vi "Setup Motors.vi"   [LabVIEW 2014]
uses:
  <vilib>/Rock Robotics/SystemInterfaces/DIO/FPGA_DIOPWMChannel.ctl
  <vilib>/Rock Robotics/WPI/Joystick/WPI_JoystickDeviceEnum.ctl
  <vilib>/Rock Robotics/SystemInterfaces/Typedef/FPGA_TypedefDigitalModule.ctl
  <vilib>/Rock Robotics/SystemInterfaces/Typedef/FPGA_TypedefAnalogModule.ctl
  <vilib>/Rock Robotics/SystemInterfaces/AI/FPGA_AIChannel.ctl
  <vilib>/Rock Robotics/WPI/Solenoid/WPI_SolenoidChannel.ctl
  <vilib>/Rock Robotics/SystemInterfaces/AI/FPGA_AIGyroChannel.ctl
  <vilib>/Rock Robotics/SystemInterfaces/Typedef/FPGA_TypedefAnalogModuleForGyro.ctl
  <vilib>/Rock Robotics/SystemInterfaces/DIO/FPGA_DIOChannel.ctl
  <vilib>/Rock Robotics/WPI/SafetyOutput/WPI_SafetyOutputConfigMenu.ctl
  <vilib>/Rock Robotics/WPI/MotorControl/WPI_MotorControlOpen Jaguar.vi
  <vilib>/Rock Robotics/WPI/MotorControl/WPI_MotorControlOpen Talon.vi
  <vilib>/Rock Robotics/WPI/Solenoid/WPI_SolenoidOpenSingle.vi
  <vilib>/Rock Robotics/WPI/Switch/WPI_SwitchOpenLimit.vi
  <vilib>/Rock Robotics/WPI/Counter/WPI_CounterDigitalInputToDigitalSource.vi
  <vilib>/Rock Robotics/WPI/Counter/WPI_CounterOpen UpDown Mode.vi
  Global Variables.vi
types:
  T1 = typedef "FPGA_DIOChannel.ctl" = enum8{"DIO 0", "DIO 1", "DIO 2", "DIO 3", "DIO 4", "DIO 5", "DIO 6", "DIO 7", "DIO 8", "DIO 9", "DIO MXP 0", "DIO MXP 1", "DIO MXP 2", "DIO MXP 3", "DIO MXP 4", "DIO MXP 5", "DIO MXP 6", "DIO MXP 7", "DIO MXP 8", "DIO MXP 9", "DIO MXP 10", "DIO MXP 11", "DIO MXP 12", "DIO MXP 13", "DIO MXP 14", "DIO MXP 15", "Invalid"}
  T2 = typedef "WPI_SafetyOutputConfigMenu.ctl" = enum16{"Enable", "Disable"}
  T3 = typedef "FPGA_TypedefDigitalModule.ctl" = enum16{"Controller 1"}
  T4 = typedef "FPGA_TypedefAnalogModuleForGyro.ctl" = enum16{"Controller 1"}
  T5 = typedef "FPGA_AIGyroChannel.ctl" = enum8{"AI 0", "AI 1", "Invalid"}
  T6 = typedef "WPI_SolenoidChannel.ctl" = enum8{"Solenoid 0", "Solenoid 1", "Solenoid 2", "Solenoid 3", "Solenoid 4", "Solenoid 5", "Solenoid 6", "Solenoid 7", "Invalid"}
  T7 = typedef "FPGA_DIOPWMChannel.ctl" = enum8{"PWM 0", "PWM 1", "PWM 2", "PWM 3", "PWM 4", "PWM 5", "PWM 6", "PWM 7", "PWM 8", "PWM 9", "PWM MXP 0", "PWM MXP 1", "PWM MXP 2", "PWM MXP 3", "PWM MXP 4", "PWM MXP 5", "PWM MXP 6", "PWM MXP 7", "PWM MXP 8", "PWM MXP 9", "Invalid"}
  T8 = typedef "FPGA_AIChannel.ctl" = enum8{"AI 0", "AI 1", "AI 2", "AI 3", "AI MXP 0", "AI MXP 1", "AI MXP 2", "AI MXP 3", "Invalid"}
  T9 = typedef "FPGA_TypedefAnalogModule.ctl" = enum16{"Controller 1"}
  T10 = typedef "WPI_JoystickDeviceEnum.ctl" = enum16{"USB 0", "USB 1", "USB 2", "USB 3", "USB 4", "USB 5"}
  T11 = typedef "WPI_MotorControlDeviceRef.ctl" = cluster{"DeviceStatus":errorcluster, "Type":T12, "PWM":cluster{"Controller":T3, "PWM Channel":T7, "DeadBand":T13}, "CAN":cluster{"Device Number":u8, "Control Mode":T14, "Semaphore":T15, "Max Vout":dbl, "TalonSRX Control Mode":T16}, "Invert":bool, "TransformRef":T17, "InvTransformRef":T17}
  T12 = typedef "WPI_MotorControlType.ctl" = enum16{"PWM", "CAN", "CANTalonSRX"}
  T13 = typedef "WPI_PWMDeadband.ctl" = cluster{"Name":string, "maxPositivePwm":i32, "minPositivePwm":i32, "centerPwm":i32, "maxNegativePwm":i32, "minNegativePwm":i32, "angularRange":u16}
  T14 = typedef "WPI_CANJaguar_ControlMode.ctl" = enum8{"Percent VBus", "Current", "Speed", "Position", "Voltage"}
  T15 = typedef "Semaphore RefNum" = refnum<k1>
  T16 = typedef "WPI_CANTalonSRX_APIControlMode.ctl" = enum8{"Percent VBus", "Speed", "Position", "Slave", "Unchanged / Invalid"}
  T17 = typedef "WPI_PWMTransform_ConPane.ctl" = refnum<vi>
  T18 = typedef "WPI_GyroDevRef.ctl" = cluster{"DevStatus":errorcluster, "Analog Module":T9, "Analog Channel":T8, "Offset":dbl, "Gain (VoltsPerDegree/Second)":dbl}
  T19 = typedef "WPI_SolenoidDevRef.ctl" = cluster{"DevStatus":errorcluster, "Pneumatics Control Module":u8, "Forward Solenoid Channel":T6, "Reverse Solenoid Channel":T6}
  T20 = typedef "WPI_SwitchDevRef.ctl" = cluster{"DevStatus":errorcluster, "DIO Channel":T1, "Controller":T3, "CntIndex":T21, "Normally Closed":bool}
  T21 = typedef "FPGA_CounterCtrSystemIndex.ctl" = enum8{"Ctr 0", "Ctr 1", "Ctr 2", "Ctr 3", "Ctr 4", "Ctr 5", "Ctr 6", "Ctr 7", "Invalid"}
  T22 = typedef "WPI_AnalogChannelDevRef.ctl" = cluster{"DevStatus":errorcluster, "Controller":T9, "Analog Channel":T8}
  T23 = typedef "WPI_DigitalInputDevRef.ctl" = cluster{"DevStatus":errorcluster, "DIO Channel":T1, "Controller":T3}
  T24 = typedef "FPGA_CounterEncoderSourceConvertionLVSourceType.ctl" = cluster{"DevStatus":errorcluster, "AnalogTriggerMode?":bool, "DigitalMode":cluster{"Controller":T3, "DIO Channel":T25}, "AnalogTriggerMode":cluster{"AnalogTriggerIndex":T26, "OutputType":T27}}
  T25 = typedef "FPGA_DIODigitalSourceChannel.ctl" = enum8{"DIO 0", "DIO 1", "DIO 2", "DIO 3", "DIO 4", "DIO 5", "DIO 6", "DIO 7", "DIO 8", "DIO 9", "DIO MXP 0", "DIO MXP 1", "DIO MXP 2", "DIO MXP 3", "DIO MXP 4", "DIO MXP 5", "DIO MXP 6", "DIO MXP 7", "DIO MXP 8", "DIO MXP 9", "DIO MXP 10", "DIO MXP 11", "DIO MXP 12", "DIO MXP 13", "DIO MXP 14", "DIO MXP 15", "Disabled"}
  T26 = typedef "FPGA_AnalogTriggerIndex.ctl" = enum8{"Trig 0", "Trig 1", "Trig 2", "Trig 3", "Trig 4", "Trig 5", "Trig 6", "Trig 7", "Invalid"}
  T27 = typedef "FPGA_AnalogTriggerOutType.ctl" = enum16{"InWindow", "TriggerState", "Rising", "Falling"}
  T28 = typedef "WPI_EncoderDevRef.ctl" = cluster{"DevStatus":errorcluster, "EncoderIndex":T29, "CounterIndex":T21, "DistancePerCount":dbl, "Decoding Type":T30}
  T29 = typedef "FPGA_EncoderIdx.ctl" = enum8{"Enc 0", "Enc 1", "Enc 2", "Enc 3", "Enc 4", "Enc 5", "Enc 6", "Enc 7", "Invalid"}
  T30 = typedef "WPI_EncoderType.ctl" = enum16{"1x", "2x", "4x"}
  T31 = typedef "WPI_CounterDevRef.ctl" = cluster{"DevStatus":errorcluster, "CntIndex":T21}
  T32 = typedef "WPI_JoystickDevRef.ctl" = cluster{"Device":T10}
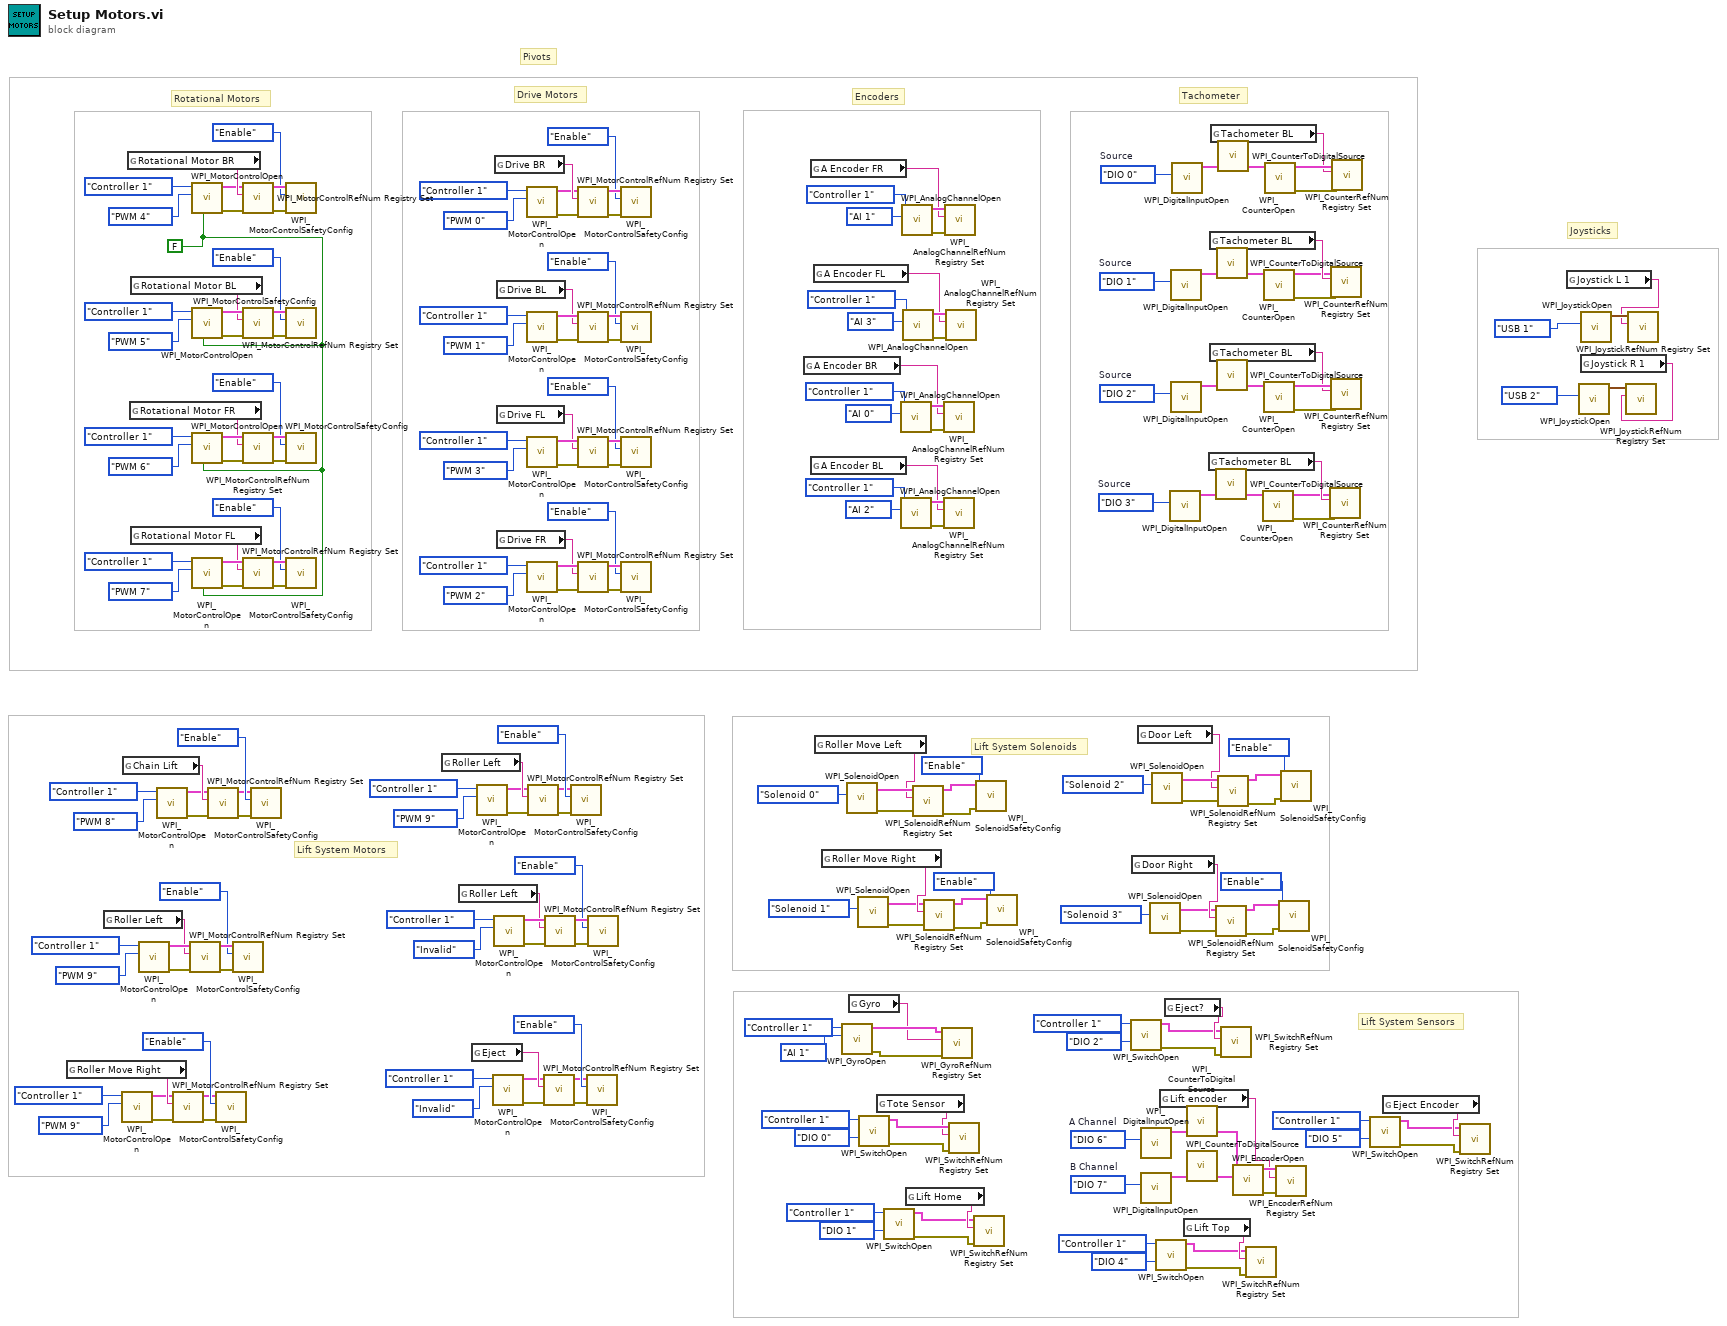
[diagram p0: block diagram]
diagram:
  w2 = FPGA_DIOChannel."DIO 3"  # Source
  w11 = FPGA_DIOChannel."DIO 2"  # Source
  w14 = FPGA_DIOChannel."DIO 1"  # Source
  w23 = FPGA_DIOChannel."DIO 0"  # Source
  w25 = FALSE ("Invert")
  w34 = FPGA_DIOChannel."DIO 7"  # B Channel
  w33 = FPGA_DIOChannel."DIO 6"  # A Channel
  # "Tachometer"
  # "Lift System Sensors"
  # "Lift System Solenoids"
  # "Lift System Motors"
  # "Encoders"
  # "Joysticks"
  # "Pivots"
  # "Rotational Motors"
  # "Drive Motors"
  n1 = global read "Global Variables.vi" "Roller Move Right"() -> (w123:string)
  n2 = global read "Global Variables.vi" "Roller Left"() -> (w126:string)
  n3 = call-poly <vilib>:"WPI_MotorControlOpen.vi"("PWM Channel"=FPGA_DIOPWMChannel."PWM 9", "Controller"=FPGA_TypedefDigitalModule."Controller 1") -> ("error out"=w118:errorcluster, "MotorControlDeviceRef"=w117:T11)  [unwired: 8 in]
  n4 = global read "Global Variables.vi" "Chain Lift"() -> (w139:string)
  n5 = global read "Global Variables.vi" "Rotational Motor BR"() -> (w193:string)
  n6 = global read "Global Variables.vi" "Rotational Motor FR"() -> (w167:string)
  n7 = global read "Global Variables.vi" "Rotational Motor BL"() -> (w168:string)
  n8 = global read "Global Variables.vi" "Rotational Motor FL"() -> (w166:string)
  n9 = call-poly <vilib>:"WPI_MotorControlOpen.vi"("PWM Channel"=FPGA_DIOPWMChannel."PWM 9", "Controller"=FPGA_TypedefDigitalModule."Controller 1") -> ("error out"=w131:errorcluster, "MotorControlDeviceRef"=w132:T11)  [unwired: 8 in]
  n10 = call-poly <vilib>:"WPI_MotorControlOpen.vi"("PWM Channel"=FPGA_DIOPWMChannel."PWM 8", "Controller"=FPGA_TypedefDigitalModule."Controller 1") -> ("error out"=w134:errorcluster, "MotorControlDeviceRef"=w133:T11)  [unwired: 8 in]
  n11 = call <vilib>:"WPI_MotorControlRefNum Registry Set.vi"("error in (no error)"=w118, "refnum name"=w123, "MotorControlDevRef"=w117) -> ("error out"=w120:errorcluster, "MotorControlDevRef"=w119:T11)  [unwired: 7 in]
  n12 = call <vilib>:"WPI_MotorControlRefNum Registry Set.vi"("error in (no error)"=w131, "refnum name"=w126, "MotorControlDevRef"=w132) -> ("error out"=w129:errorcluster, "MotorControlDevRef"=w130:T11)  [unwired: 7 in]
  n13 = call-poly <vilib>:"WPI_MotorControlOpen.vi"("Invert"=w25, "PWM Channel"=FPGA_DIOPWMChannel."PWM 4", "Controller"=FPGA_TypedefDigitalModule."Controller 1") -> ("error out"=w191:errorcluster, "MotorControlDeviceRef"=w192:T11)  [unwired: 7 in]
  n14 = call-poly <vilib>:"WPI_MotorControlOpen.vi"("Invert"=w25, "PWM Channel"=FPGA_DIOPWMChannel."PWM 5", "Controller"=FPGA_TypedefDigitalModule."Controller 1") -> ("error out"=w185:errorcluster, "MotorControlDeviceRef"=w186:T11)  [unwired: 7 in]
  n15 = call-poly <vilib>:"WPI_MotorControlOpen.vi"("Invert"=w25, "PWM Channel"=FPGA_DIOPWMChannel."PWM 6", "Controller"=FPGA_TypedefDigitalModule."Controller 1") -> ("error out"=w179:errorcluster, "MotorControlDeviceRef"=w180:T11)  [unwired: 7 in]
  n16 = call-poly <vilib>:"WPI_MotorControlOpen.vi"("Invert"=w25, "PWM Channel"=FPGA_DIOPWMChannel."PWM 7", "Controller"=FPGA_TypedefDigitalModule."Controller 1") -> ("error out"=w173:errorcluster, "MotorControlDeviceRef"=w174:T11)  [unwired: 7 in]
  n17 = call <vilib>:"WPI_MotorControlRefNum Registry Set.vi"("error in (no error)"=w134, "refnum name"=w139, "MotorControlDevRef"=w133) -> ("error out"=w136:errorcluster, "MotorControlDevRef"=w135:T11)  [unwired: 7 in]
  n18 = call <vilib>:"WPI_MotorControlSafetyConfig.vi"("error in (no error)"=w120, "mode"=WPI_SafetyOutputConfigMenu."Enable", "MotorControlDevRef"=w119) -> ()  [unwired: 7 in, 2 out]
  n19 = call <vilib>:"WPI_MotorControlSafetyConfig.vi"("error in (no error)"=w129, "mode"=WPI_SafetyOutputConfigMenu."Enable", "MotorControlDevRef"=w130) -> ()  [unwired: 7 in, 2 out]
  n20 = call <vilib>:"WPI_MotorControlRefNum Registry Set.vi"("error in (no error)"=w191, "refnum name"=w193, "MotorControlDevRef"=w192) -> ("error out"=w189:errorcluster, "MotorControlDevRef"=w190:T11)  [unwired: 7 in]
  n21 = call <vilib>:"WPI_MotorControlRefNum Registry Set.vi"("error in (no error)"=w185, "refnum name"=w168, "MotorControlDevRef"=w186) -> ("error out"=w183:errorcluster, "MotorControlDevRef"=w184:T11)  [unwired: 7 in]
  n22 = call <vilib>:"WPI_MotorControlRefNum Registry Set.vi"("error in (no error)"=w179, "refnum name"=w167, "MotorControlDevRef"=w180) -> ("error out"=w177:errorcluster, "MotorControlDevRef"=w178:T11)  [unwired: 7 in]
  n23 = call <vilib>:"WPI_MotorControlRefNum Registry Set.vi"("error in (no error)"=w173, "refnum name"=w166, "MotorControlDevRef"=w174) -> ("error out"=w171:errorcluster, "MotorControlDevRef"=w172:T11)  [unwired: 7 in]
  n24 = call <vilib>:"WPI_MotorControlSafetyConfig.vi"("error in (no error)"=w136, "mode"=WPI_SafetyOutputConfigMenu."Enable", "MotorControlDevRef"=w135) -> ()  [unwired: 7 in, 2 out]
  n25 = call <vilib>:"WPI_MotorControlSafetyConfig.vi"("error in (no error)"=w189, "mode"=WPI_SafetyOutputConfigMenu."Enable", "MotorControlDevRef"=w190) -> ()  [unwired: 7 in, 2 out]
  n26 = call <vilib>:"WPI_MotorControlSafetyConfig.vi"("error in (no error)"=w183, "mode"=WPI_SafetyOutputConfigMenu."Enable", "MotorControlDevRef"=w184) -> ()  [unwired: 7 in, 2 out]
  n27 = call <vilib>:"WPI_MotorControlSafetyConfig.vi"("error in (no error)"=w177, "mode"=WPI_SafetyOutputConfigMenu."Enable", "MotorControlDevRef"=w178) -> ()  [unwired: 7 in, 2 out]
  n28 = call <vilib>:"WPI_MotorControlSafetyConfig.vi"("error in (no error)"=w171, "mode"=WPI_SafetyOutputConfigMenu."Enable", "MotorControlDevRef"=w172) -> ()  [unwired: 7 in, 2 out]
  n29 = global read "Global Variables.vi" "Roller Left"() -> (w115:string)
  n30 = global read "Global Variables.vi" "Roller Left"() -> (w102:string)
  n31 = global read "Global Variables.vi" "Eject"() -> (w99:string)
  n32 = call-poly <vilib>:"WPI_MotorControlOpen.vi"("PWM Channel"=FPGA_DIOPWMChannel."PWM 9", "Controller"=FPGA_TypedefDigitalModule."Controller 1") -> ("error out"=w110:errorcluster, "MotorControlDeviceRef"=w109:T11)  [unwired: 8 in]
  n33 = call-poly <vilib>:"WPI_MotorControlOpen.vi"("PWM Channel"=FPGA_DIOPWMChannel."Invalid", "Controller"=FPGA_TypedefDigitalModule."Controller 1") -> ("error out"=w94:errorcluster, "MotorControlDeviceRef"=w93:T11)  [unwired: 8 in]
  n34 = call-poly <vilib>:"WPI_MotorControlOpen.vi"("PWM Channel"=FPGA_DIOPWMChannel."Invalid", "Controller"=FPGA_TypedefDigitalModule."Controller 1") -> ("error out"=w107:errorcluster, "MotorControlDeviceRef"=w108:T11)  [unwired: 8 in]
  n35 = global read "Global Variables.vi" "Drive BR"() -> (w230:string)
  n36 = global read "Global Variables.vi" "Drive BL"() -> (w205:string)
  n37 = global read "Global Variables.vi" "Drive FL"() -> (w204:string)
  n38 = global read "Global Variables.vi" "Drive FR"() -> (w203:string)
  n39 = call-poly <vilib>:"WPI_MotorControlOpen.vi"("PWM Channel"=FPGA_DIOPWMChannel."PWM 0", "Controller"=FPGA_TypedefDigitalModule."Controller 1") -> ("error out"=w228:errorcluster, "MotorControlDeviceRef"=w229:T11)  [unwired: 8 in]
  n40 = call-poly <vilib>:"WPI_MotorControlOpen.vi"("PWM Channel"=FPGA_DIOPWMChannel."PWM 1", "Controller"=FPGA_TypedefDigitalModule."Controller 1") -> ("error out"=w222:errorcluster, "MotorControlDeviceRef"=w223:T11)  [unwired: 8 in]
  n41 = call-poly <vilib>:"WPI_MotorControlOpen.vi"("PWM Channel"=FPGA_DIOPWMChannel."PWM 3", "Controller"=FPGA_TypedefDigitalModule."Controller 1") -> ("error out"=w216:errorcluster, "MotorControlDeviceRef"=w217:T11)  [unwired: 8 in]
  n42 = call-poly <vilib>:"WPI_MotorControlOpen.vi"("PWM Channel"=FPGA_DIOPWMChannel."PWM 2", "Controller"=FPGA_TypedefDigitalModule."Controller 1") -> ("error out"=w210:errorcluster, "MotorControlDeviceRef"=w211:T11)  [unwired: 8 in]
  n43 = call <vilib>:"WPI_MotorControlRefNum Registry Set.vi"("error in (no error)"=w110, "refnum name"=w115, "MotorControlDevRef"=w109) -> ("error out"=w112:errorcluster, "MotorControlDevRef"=w111:T11)  [unwired: 7 in]
  n44 = call <vilib>:"WPI_MotorControlRefNum Registry Set.vi"("error in (no error)"=w94, "refnum name"=w99, "MotorControlDevRef"=w93) -> ("error out"=w96:errorcluster, "MotorControlDevRef"=w95:T11)  [unwired: 7 in]
  n45 = call <vilib>:"WPI_MotorControlRefNum Registry Set.vi"("error in (no error)"=w107, "refnum name"=w102, "MotorControlDevRef"=w108) -> ("error out"=w105:errorcluster, "MotorControlDevRef"=w106:T11)  [unwired: 7 in]
  n46 = call <vilib>:"WPI_MotorControlSafetyConfig.vi"("error in (no error)"=w112, "mode"=WPI_SafetyOutputConfigMenu."Enable", "MotorControlDevRef"=w111) -> ()  [unwired: 7 in, 2 out]
  n47 = call <vilib>:"WPI_MotorControlRefNum Registry Set.vi"("error in (no error)"=w228, "refnum name"=w230, "MotorControlDevRef"=w229) -> ("error out"=w226:errorcluster, "MotorControlDevRef"=w227:T11)  [unwired: 7 in]
  n48 = call <vilib>:"WPI_MotorControlRefNum Registry Set.vi"("error in (no error)"=w222, "refnum name"=w205, "MotorControlDevRef"=w223) -> ("error out"=w220:errorcluster, "MotorControlDevRef"=w221:T11)  [unwired: 7 in]
  n49 = call <vilib>:"WPI_MotorControlRefNum Registry Set.vi"("error in (no error)"=w216, "refnum name"=w204, "MotorControlDevRef"=w217) -> ("error out"=w214:errorcluster, "MotorControlDevRef"=w215:T11)  [unwired: 7 in]
  n50 = call <vilib>:"WPI_MotorControlRefNum Registry Set.vi"("error in (no error)"=w210, "refnum name"=w203, "MotorControlDevRef"=w211) -> ("error out"=w208:errorcluster, "MotorControlDevRef"=w209:T11)  [unwired: 7 in]
  n51 = call <vilib>:"WPI_MotorControlSafetyConfig.vi"("error in (no error)"=w96, "mode"=WPI_SafetyOutputConfigMenu."Enable", "MotorControlDevRef"=w95) -> ()  [unwired: 7 in, 2 out]
  n52 = call <vilib>:"WPI_MotorControlSafetyConfig.vi"("error in (no error)"=w105, "mode"=WPI_SafetyOutputConfigMenu."Enable", "MotorControlDevRef"=w106) -> ()  [unwired: 7 in, 2 out]
  n53 = call <vilib>:"WPI_MotorControlSafetyConfig.vi"("error in (no error)"=w226, "mode"=WPI_SafetyOutputConfigMenu."Enable", "MotorControlDevRef"=w227) -> ()  [unwired: 7 in, 2 out]
  n54 = call <vilib>:"WPI_MotorControlSafetyConfig.vi"("error in (no error)"=w220, "mode"=WPI_SafetyOutputConfigMenu."Enable", "MotorControlDevRef"=w221) -> ()  [unwired: 7 in, 2 out]
  n55 = call <vilib>:"WPI_MotorControlSafetyConfig.vi"("error in (no error)"=w214, "mode"=WPI_SafetyOutputConfigMenu."Enable", "MotorControlDevRef"=w215) -> ()  [unwired: 7 in, 2 out]
  n56 = call <vilib>:"WPI_MotorControlSafetyConfig.vi"("error in (no error)"=w208, "mode"=WPI_SafetyOutputConfigMenu."Enable", "MotorControlDevRef"=w209) -> ()  [unwired: 7 in, 2 out]
  n57 = global read "Global Variables.vi" "A Encoder BR"() -> (w142:string)
  n58 = global read "Global Variables.vi" "A Encoder FR"() -> (w144:string)
  n59 = global read "Global Variables.vi" "A Encoder BL"() -> (w143:string)
  n60 = global read "Global Variables.vi" "A Encoder FL"() -> (w141:string)
  n61 = global read "Global Variables.vi" "Roller Move Left"() -> (w87:string)
  n62 = global read "Global Variables.vi" "Roller Move Right"() -> (w86:string)
  n63 = call <vilib>:"WPI_GyroOpen.vi"("Analog Channel"=FPGA_AIGyroChannel."AI 1", "Controller"=FPGA_TypedefAnalogModuleForGyro."Controller 1") -> ("error out"=w67:errorcluster, "GyroDevRef"=w68:T18)  [unwired: 7 in, 1 out]
  n64 = call-poly <vilib>:"WPI_SolenoidOpen.vi"("Solenoid Channel"=WPI_SolenoidChannel."Solenoid 0") -> ("error out"=w89:errorcluster, "SolenoidDevRef"=w90:T19)  [unwired: 9 in]
  n65 = global read "Global Variables.vi" "Gyro"() -> (w64:string)
  n66 = call-poly <vilib>:"WPI_SolenoidOpen.vi"("Solenoid Channel"=WPI_SolenoidChannel."Solenoid 1") -> ("error out"=w84:errorcluster, "SolenoidDevRef"=w83:T19)  [unwired: 9 in]
  n67 = call-poly <vilib>:"WPI_SwitchOpen.vi"("DIO Channel"=FPGA_DIOChannel."DIO 0", "Controller"=FPGA_TypedefDigitalModule."Controller 1") -> ("error out"=w62:errorcluster, "SwitchDevRef"=w63:T20)  [unwired: 8 in]
  n68 = global read "Global Variables.vi" "Tote Sensor"() -> (w59:string)
  n69 = call-poly <vilib>:"WPI_SwitchOpen.vi"("DIO Channel"=FPGA_DIOChannel."DIO 1", "Controller"=FPGA_TypedefDigitalModule."Controller 1") -> ("error out"=w55:errorcluster, "SwitchDevRef"=w54:T20)  [unwired: 8 in]
  n70 = call <vilib>:"WPI_AnalogChannelOpen.vi"("Analog Channel"=FPGA_AIChannel."AI 0", "Controller"=FPGA_TypedefAnalogModule."Controller 1") -> ("error out"=w151:errorcluster, "AIDeviceRef"=w152:T22)  [unwired: 8 in]
  n71 = call <vilib>:"WPI_AnalogChannelOpen.vi"("Analog Channel"=FPGA_AIChannel."AI 2", "Controller"=FPGA_TypedefAnalogModule."Controller 1") -> ("error out"=w147:errorcluster, "AIDeviceRef"=w148:T22)  [unwired: 8 in]
  n72 = call <vilib>:"WPI_AnalogChannelOpen.vi"("Analog Channel"=FPGA_AIChannel."AI 1", "Controller"=FPGA_TypedefAnalogModule."Controller 1") -> ("error out"=w159:errorcluster, "AIDeviceRef"=w160:T22)  [unwired: 8 in]
  n73 = call <vilib>:"WPI_AnalogChannelOpen.vi"("Analog Channel"=FPGA_AIChannel."AI 3", "Controller"=FPGA_TypedefAnalogModule."Controller 1") -> ("error out"=w155:errorcluster, "AIDeviceRef"=w156:T22)  [unwired: 8 in]
  n74 = global read "Global Variables.vi" "Lift Home"() -> (w58:string)
  n75 = call <vilib>:"WPI_SolenoidRefNum Registry Set.vi"("error in (no error)"=w89, "refnum name"=w87, "SolenoidDevRef"=w90) -> ("error out"=w91:errorcluster, "SolenoidDevRef"=w92:T19)  [unwired: 7 in]
  n76 = call <vilib>:"WPI_SolenoidRefNum Registry Set.vi"("error in (no error)"=w84, "refnum name"=w86, "SolenoidDevRef"=w83) -> ("error out"=w82:errorcluster, "SolenoidDevRef"=w81:T19)  [unwired: 7 in]
  n77 = call <vilib>:"WPI_GyroRefNum Registry Set.vi"("error in (no error)"=w67, "refnum name"=w64, "GyroDevRef"=w68) -> ()  [unwired: 7 in, 2 out]
  n78 = call <vilib>:"WPI_AnalogChannelRefNum Registry Set.vi"("error in (no error)"=w151, "refnum name"=w142, "AIDeviceRef"=w152) -> ()  [unwired: 7 in, 2 out]
  n79 = call <vilib>:"WPI_AnalogChannelRefNum Registry Set.vi"("error in (no error)"=w147, "refnum name"=w143, "AIDeviceRef"=w148) -> ()  [unwired: 7 in, 2 out]
  n80 = call <vilib>:"WPI_AnalogChannelRefNum Registry Set.vi"("error in (no error)"=w159, "refnum name"=w144, "AIDeviceRef"=w160) -> ()  [unwired: 7 in, 2 out]
  n81 = call <vilib>:"WPI_AnalogChannelRefNum Registry Set.vi"("error in (no error)"=w155, "refnum name"=w141, "AIDeviceRef"=w156) -> ()  [unwired: 7 in, 2 out]
  n82 = call <vilib>:"WPI_SwitchRefNum Registry Set.vi"("error in (no error)"=w62, "refnum name"=w59, "SwitchDevRef"=w63) -> ()  [unwired: 7 in, 2 out]
  n83 = call <vilib>:"WPI_SwitchRefNum Registry Set.vi"("error in (no error)"=w55, "refnum name"=w58, "SwitchDevRef"=w54) -> ()  [unwired: 7 in, 2 out]
  n84 = call <vilib>:"WPI_SolenoidSafetyConfig.vi"("error in (no error)"=w91, "mode"=WPI_SafetyOutputConfigMenu."Enable", "SolenoidDevRef"=w92) -> ()  [unwired: 7 in, 2 out]
  n85 = call <vilib>:"WPI_SolenoidSafetyConfig.vi"("error in (no error)"=w82, "mode"=WPI_SafetyOutputConfigMenu."Enable", "SolenoidDevRef"=w81) -> ()  [unwired: 7 in, 2 out]
  n86 = call-poly <vilib>:"WPI_SwitchOpen.vi"("DIO Channel"=FPGA_DIOChannel."DIO 2", "Controller"=FPGA_TypedefDigitalModule."Controller 1") -> ("error out"=w45:errorcluster, "SwitchDevRef"=w44:T20)  [unwired: 8 in]
  n87 = global read "Global Variables.vi" "Door Right"() -> (w74:string)
  n88 = global read "Global Variables.vi" "Door Left"() -> (w75:string)
  n89 = call <vilib>:"WPI_DigitalInputOpen.vi"("DIO Channel"=w33) -> ("DigitalInputDevRef"=w30:T23)  [unwired: 2 in, 8 out]
  n90 = call <vilib>:"WPI_DigitalInputOpen.vi"("DIO Channel"=w34) -> ("DigitalInputDevRef"=w31:T23)  [unwired: 2 in, 8 out]
  n91 = call-poly <vilib>:"WPI_SolenoidOpen.vi"("Solenoid Channel"=WPI_SolenoidChannel."Solenoid 3") -> ("error out"=w72:errorcluster, "SolenoidDevRef"=w71:T19)  [unwired: 9 in]
  n92 = call-poly <vilib>:"WPI_SolenoidOpen.vi"("Solenoid Channel"=WPI_SolenoidChannel."Solenoid 2") -> ("error out"=w77:errorcluster, "SolenoidDevRef"=w78:T19)  [unwired: 9 in]
  n93 = call-poly <vilib>:"WPI_SwitchOpen.vi"("DIO Channel"=FPGA_DIOChannel."DIO 4", "Controller"=FPGA_TypedefDigitalModule."Controller 1") -> ("error out"=w50:errorcluster, "SwitchDevRef"=w49:T20)  [unwired: 8 in]
  n94 = global read "Global Variables.vi" "Lift encoder"() -> (w26:string)
  n95 = global read "Global Variables.vi" "Eject?"() -> (w48:string)
  n96 = call <vilib>:"WPI_DigitalInputOpen.vi"("DIO Channel"=w2) -> ("DigitalInputDevRef"=w3:T23)  [unwired: 2 in, 8 out]
  n97 = call <vilib>:"WPI_DigitalInputOpen.vi"("DIO Channel"=w14) -> ("DigitalInputDevRef"=w15:T23)  [unwired: 2 in, 8 out]
  n98 = call <vilib>:"WPI_DigitalInputOpen.vi"("DIO Channel"=w11) -> ("DigitalInputDevRef"=w10:T23)  [unwired: 2 in, 8 out]
  n99 = call <vilib>:"WPI_DigitalInputOpen.vi"("DIO Channel"=w23) -> ("DigitalInputDevRef"=w22:T23)  [unwired: 2 in, 8 out]
  n100 = global read "Global Variables.vi" "Lift Top"() -> (w53:string)
  n101 = call-poly <vilib>:"WPI_CounterToDigitalSource.vi"("DigitalInputDevRef"=w30) -> ("Digital Source"=w29:T24)  [unwired: 6 out]
  n102 = call-poly <vilib>:"WPI_CounterToDigitalSource.vi"("DigitalInputDevRef"=w31) -> ("Digital Source"=w32:T24)  [unwired: 6 out]
  n103 = global read "Global Variables.vi" "Tachometer BL"() -> (w6:string)
  n104 = global read "Global Variables.vi" "Tachometer BL"() -> (w18:string)
  n105 = global read "Global Variables.vi" "Tachometer BL"() -> (w7:string)
  n106 = global read "Global Variables.vi" "Tachometer BL"() -> (w19:string)
  n107 = call-poly <vilib>:"WPI_CounterToDigitalSource.vi"("DigitalInputDevRef"=w3) -> ("Digital Source"=w1:T24)  [unwired: 6 out]
  n108 = call <vilib>:"WPI_SolenoidRefNum Registry Set.vi"("error in (no error)"=w72, "refnum name"=w74, "SolenoidDevRef"=w71) -> ("error out"=w70:errorcluster, "SolenoidDevRef"=w69:T19)  [unwired: 7 in]
  n109 = call-poly <vilib>:"WPI_CounterToDigitalSource.vi"("DigitalInputDevRef"=w15) -> ("Digital Source"=w13:T24)  [unwired: 6 out]
  n110 = call-poly <vilib>:"WPI_CounterToDigitalSource.vi"("DigitalInputDevRef"=w10) -> ("Digital Source"=w12:T24)  [unwired: 6 out]
  n111 = call-poly <vilib>:"WPI_CounterToDigitalSource.vi"("DigitalInputDevRef"=w22) -> ("Digital Source"=w24:T24)  [unwired: 6 out]
  n112 = call <vilib>:"WPI_SolenoidRefNum Registry Set.vi"("error in (no error)"=w77, "refnum name"=w75, "SolenoidDevRef"=w78) -> ("error out"=w79:errorcluster, "SolenoidDevRef"=w80:T19)  [unwired: 7 in]
  n113 = call <vilib>:"WPI_SwitchRefNum Registry Set.vi"("error in (no error)"=w45, "refnum name"=w48, "SwitchDevRef"=w44) -> ()  [unwired: 7 in, 2 out]
  n114 = call <vilib>:"WPI_EncoderOpen.vi"("BSource"=w32, "ASource"=w29) -> ("error out"=w28:errorcluster, "EncoderDevRef"=w27:T28)  [unwired: 6 in, 2 out]
  n115 = call <vilib>:"WPI_SwitchRefNum Registry Set.vi"("error in (no error)"=w50, "refnum name"=w53, "SwitchDevRef"=w49) -> ()  [unwired: 7 in, 2 out]
  n116 = call-poly <vilib>:"WPI_CounterOpen.vi"("Up Source"=w1) -> ("error out"=w5:errorcluster, "CounterDevRef"=w4:T31)  [unwired: 6 in, 3 out]
  n117 = call-poly <vilib>:"WPI_CounterOpen.vi"("Up Source"=w13) -> ("error out"=w17:errorcluster, "CounterDevRef"=w16:T31)  [unwired: 6 in, 3 out]
  n118 = call-poly <vilib>:"WPI_CounterOpen.vi"("Up Source"=w12) -> ("error out"=w8:errorcluster, "CounterDevRef"=w9:T31)  [unwired: 6 in, 3 out]
  n119 = call-poly <vilib>:"WPI_CounterOpen.vi"("Up Source"=w24) -> ("error out"=w20:errorcluster, "CounterDevRef"=w21:T31)  [unwired: 6 in, 3 out]
  n120 = call <vilib>:"WPI_EncoderRefNum Registry Set.vi"("error in (no error)"=w28, "refnum name"=w26, "EncoderDevRef"=w27) -> ()  [unwired: 7 in, 2 out]
  n121 = call <vilib>:"WPI_SolenoidSafetyConfig.vi"("error in (no error)"=w70, "mode"=WPI_SafetyOutputConfigMenu."Enable", "SolenoidDevRef"=w69) -> ()  [unwired: 7 in, 2 out]
  n122 = call <vilib>:"WPI_SolenoidSafetyConfig.vi"("error in (no error)"=w79, "mode"=WPI_SafetyOutputConfigMenu."Enable", "SolenoidDevRef"=w80) -> ()  [unwired: 7 in, 2 out]
  n123 = call <vilib>:"WPI_CounterRefNum Registry Set.vi"("error in (no error)"=w5, "refnum name"=w6, "CounterDevRef"=w4) -> ()  [unwired: 7 in, 2 out]
  n124 = call <vilib>:"WPI_CounterRefNum Registry Set.vi"("error in (no error)"=w17, "refnum name"=w18, "CounterDevRef"=w16) -> ()  [unwired: 7 in, 2 out]
  n125 = call <vilib>:"WPI_CounterRefNum Registry Set.vi"("error in (no error)"=w8, "refnum name"=w7, "CounterDevRef"=w9) -> ()  [unwired: 7 in, 2 out]
  n126 = call <vilib>:"WPI_CounterRefNum Registry Set.vi"("error in (no error)"=w20, "refnum name"=w19, "CounterDevRef"=w21) -> ()  [unwired: 7 in, 2 out]
  n127 = call-poly <vilib>:"WPI_SwitchOpen.vi"("DIO Channel"=FPGA_DIOChannel."DIO 5", "Controller"=FPGA_TypedefDigitalModule."Controller 1") -> ("error out"=w40:errorcluster, "SwitchDevRef"=w39:T20)  [unwired: 8 in]
  n128 = global read "Global Variables.vi" "Eject Encoder"() -> (w43:string)
  n129 = call <vilib>:"WPI_SwitchRefNum Registry Set.vi"("error in (no error)"=w40, "refnum name"=w43, "SwitchDevRef"=w39) -> ()  [unwired: 7 in, 2 out]
  n130 = global read "Global Variables.vi" "Joystick L 1"() -> (w197:string)
  n131 = call <vilib>:"WPI_JoystickOpen.vi"("JoystickDevice"=WPI_JoystickDeviceEnum."USB 2") -> ("JoystickDevRef"=w195:T32)  [unwired: 10 in]
  n132 = call <vilib>:"WPI_JoystickOpen.vi"("JoystickDevice"=WPI_JoystickDeviceEnum."USB 1") -> ("JoystickDevRef"=w198:T32)  [unwired: 10 in]
  n133 = global read "Global Variables.vi" "Joystick R 1"() -> (w194:string)
  n134 = call <vilib>:"WPI_JoystickRefNum Registry Set.vi"("refnum name"=w194, "JoystickDevRef"=w195) -> ()  [unwired: 8 in, 2 out]
  n135 = call <vilib>:"WPI_JoystickRefNum Registry Set.vi"("refnum name"=w197, "JoystickDevRef"=w198) -> ()  [unwired: 8 in, 2 out]
